vi "To Center and Span (array).vi"(5 "start/stop":T2 {"stop" min=0.0 step=10000.0 format="%.2g"; "start" min=0.0 step=10000.0 format="%.2g"}) -> (1 "center/span":T1 {"span" min=0.0 step=10000.0 format="%.2g"; "center" min=0.0 step=10000.0 format="%.2g"})   [LabVIEW 2023]
doc: "Takes two bare numbers that indicate the beginning and end of a range and returns the average (\"center\") and difference (\"span\") of the two numbers."
uses:
  FG FM sweep start stop control.ctl
  FG FM sweep center span control.ctl
  Math Operations/To Center and Span (frequency).vi
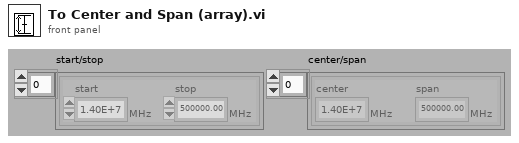
[diagram p1: front panel]
types:
  T1 = typedef "FG FM sweep center span control.ctl" = cluster{"center":dbl[unit], "span":dbl[unit]}[]
  T2 = typedef "FG FM sweep start stop control.ctl" = cluster{"start":dbl[unit], "stop":dbl[unit]}[]
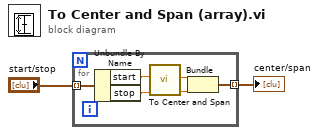
[diagram p0: block diagram]
diagram:
  n1 = for {
    tunnel: "start/stop" -> [w8] mode=indexing
    tunnel: [w3] -> w1 mode=indexing
    n2 = Unbundle By Name(w8) -> ("start"=w7:dbl[unit], "stop"=w6:dbl[unit])
    n3 = call-poly "To Center and Span.vi"("stop"=w6, "start"=w7) -> ("span"=w4:dbl[unit], "center"=w5:dbl[unit])  [unwired: 4 out]
    n4 = Bundle("center"=w5, "span"=w4) -> (w3:cluster{"center":dbl[unit], "span":dbl[unit]})  [unwired: 1 out]
  }
  "center/span" <- w1
